vi "SS2 Live_Check Gate Definition Authorizaton.vi"(8 "Error In":errorcluster, 9 "OldVal":variant, 10 "NewVal":variant, 11 "Control Refnum":refnum<vi>) -> (0 "Error Out":errorcluster, 1 "Change Accepted?":bool, 2 "NewVal":variant, 3 "Control Refnum":refnum<vi>)   [LabVIEW 2019]
uses:
  SS2 DAQ Parameters 2.ctl
  SS2 Gate Definition.ctl
  SS2 Live_Globals.vi
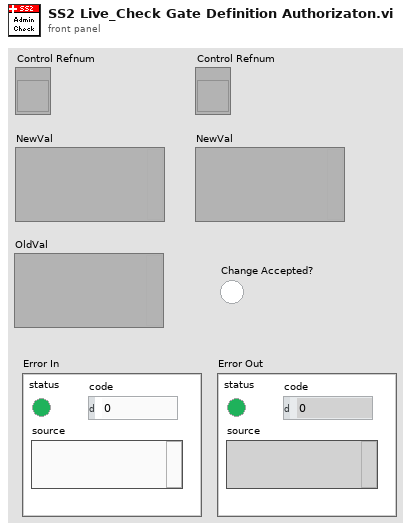
[diagram p1: front panel]
types:
  T1 = typedef "SS2 DAQ Parameters 2.ctl" = cluster{"10 bits":bool, "# Exposure Sequences":u32, "# 1-bit Frame per Gate":u32, "Gate Shift":u32, "# Gates per Set":u32, "# Sets":u32, "Laser Period":dbl[unit], "Gate Offset":u32, "Auto-adjust Gate Offset":bool, "Gate Definition":T2}
  T2 = typedef "SS2 Gate Definition.ctl" = cluster{"gs_psincdec_0":u32, "gs_psincdec_1":u32, "gs_psincdec_2":u32, "gs_psincdec_3":u32, "gs_no_shift_adj_1":u32, "gs_no_shift_adj_2":u32, "gs_no_shift_adj_3":u32}
  T3 = cluster{"10 bits":bool, "# Exposure Sequences":bool, "# 1-bit Frame per Gate":bool, "Gate Shift":bool, "# Gates per Set":bool, "# Sets":bool, "Laser Period":bool, "Gate Offset":bool, "Auto-adjust Gate Offset":bool, "Gate Definition":cluster{"gs_psincdec_0":bool, "gs_psincdec_1":bool, "gs_psincdec_2":bool, "gs_psincdec_3":bool, "gs_no_shift_adj_1":bool, "gs_no_shift_adj_2":bool, "gs_no_shift_adj_3":bool}}
  T4 = cluster{"gs_psincdec_0":bool, "gs_psincdec_1":bool, "gs_psincdec_2":bool, "gs_psincdec_3":bool, "gs_no_shift_adj_1":bool, "gs_no_shift_adj_2":bool, "gs_no_shift_adj_3":bool}
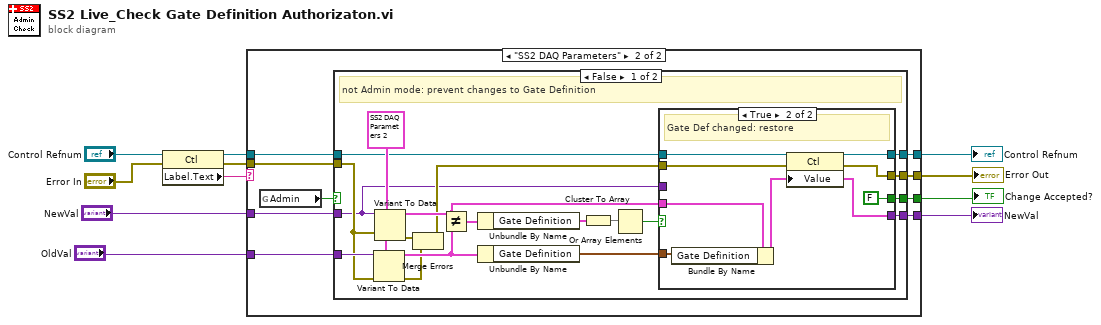
[diagram p0: block diagram]
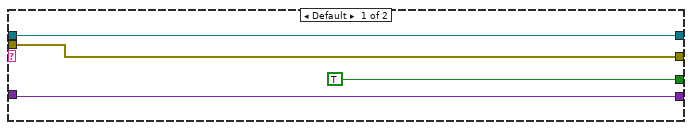
[diagram p2: hidden frame]
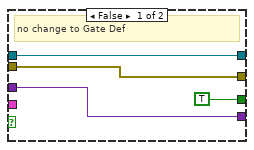
[diagram p3: hidden frame]
diagram:
  n1 = property class="Ctl"(reference="Control Refnum", error in="Error In") -> (reference out=w8:refnum<vi>, error out=w3:errorcluster, "Label.Text"=w9:string)
  n2 = case shown="\"SS2 DAQ Parameters\"" w9 {
    tunnel: w8 -> [w15 w23]
    tunnel: [w15 w22] -> w7
    tunnel: "NewVal" -> [w14 w21]
    tunnel: [w14 w20] -> w5
    tunnel: [w13 w18] -> w4
    tunnel: w3 -> [w13 w17]
    tunnel: [TRUE ("Change Accepted?") w19] -> w2
    tunnel: "OldVal" -> [_ w16]
    frame Default {
    }
    frame "SS2 DAQ Parameters" {
      n3 = global read "SS2 Live_Globals.vi" "Admin"() -> (w24:bool)
      n4 = case shown="False" w24 {
        selector: w24 -> [_ w57]
        tunnel: w23 -> [w33 w59]
        tunnel: [w32 w59] -> w22
        tunnel: w21 -> [w26 w58]
        tunnel: [w25 w58] -> w20
        tunnel: [w27 w57] -> w19
        tunnel: [w28 w56] -> w18
        tunnel: w17 -> [w42 w56]
        tunnel: w16 -> [w43 _]
        frame False {
          w41 = T1 {"10 bits"=FALSE, "# Exposure Sequences"=0, "# 1-bit Frame per Gate"=255, "Gate Shift"=0, "# Gates per Set"=0, "# Sets"=1, "Laser Period"=0.0, "Gate Offset"=0, "Auto-adjust Gate Offset"=FALSE, "Gate Definition"={"gs_psincdec_0"=0, "gs_psincdec_1"=0, "gs_psincdec_2"=0, "gs_psincdec_3"=0, "gs_no_shift_adj_1"=0, "gs_no_shift_adj_2"=0, "gs_no_shift_adj_3"=0}} ("SS2 DAQ Parameters")
          # "not Admin mode: prevent changes to Gate Definition"
          n5 = Variant To Data(error in=w42, type=w41, Variant=w43) -> (data=w37:T1, error out=w30:errorcluster)
          n6 = Variant To Data(error in=w42, type=w41, Variant=w26) -> (data=w35:T1, error out=w31:errorcluster)
          n7 = Merge Errors(w31, w30) -> (w29:errorcluster)
          n8 = Not Equal?(x=w35, y=w37) -> (x != y?=w40:T3)
          n9 = Unbundle By Name(w40) -> ("Gate Definition"=w39:T4)
          n10 = Unbundle By Name(w37) -> ("Gate Definition"=w34:T2)
          n11 = Cluster To Array(cluster=w39) -> (array=w38:bool[])
          n12 = Or Array Elements(Boolean array=w38) -> (logical OR=w36:bool)
          n13 = case shown="True" w36 {
            tunnel: w35 -> [_ w55]
            tunnel: w34 -> [_ w54]
            tunnel: w33 -> [w47 w53]
            tunnel: [w47 w52] -> w32
            tunnel: w29 -> [w46 w51]
            tunnel: [w46 w50] -> w28
            tunnel: [TRUE FALSE] -> w27
            tunnel: w26 -> [w44 _]
            tunnel: [w44 w49] -> w25
            frame False {
              # "no change to Gate Def"
            }
            frame True {
              # "Gate Def changed: restore"
              n14 = Bundle By Name(cluster=w55, "Gate Definition"=w54) -> (w49:T1)
              n15 = property class="Ctl"(reference=w53, error in=w51, "Value"=w49) -> (reference out=w52:refnum<vi>, error out=w50:errorcluster)
            }
          }
        }
        frame True {
          # "Admin mode: changes OK"
        }
      }
    }
  }
  "NewVal" <- w5
  "Control Refnum" <- w7
  "Error Out" <- w4
  "Change Accepted?" <- w2
